vi "Generate Patch Seq Img Core.vi"(0 "tdms file ref":refnum<k34>, 1 "Channel to process":enum16{"Red", "Green"}(ring), 5 "All header parameters":T1={"LOGIN"={"User"="Olympus  20X", "Profile"="", "Software Version"="", "Experiment Date Time"=timestamp(0 s since 1904-01-01)}, "GLOBAL PARAMETERS"={"MicroscopeID"="", "Microscope Type"="", "Objective"="", "Field of View (um)"=0.0, "Fill time (us)"=0.0, "Experiment Type"=enum."In vivo", "Stimuli Trigger"=FALSE, "Speed Logging"=FALSE}, "IMAGING MODES"={"Time Series"=FALSE, "Motor Zstack"=FALSE, "AOL Zstack"=FALSE, "Functional Imaging"=FALSE, "Volume Imaging"=FALSE}, "TIME SERIES"={"Basic Image meta data"={"Wavelength (nm)"=0.0, "# averaged frames"=0.0, "laser power (%)"=0.0, "Pockels"=0.0, "pixel dwell time (us)"=0.0, "pmt 1"=0.0, "pmt 2"=0.0, "back apperture"=0.0, "zoom"=0.0, "field of view"=0.0, "Frame Size"=200, "AOL x centre"=0.0, "AOL y centre"=0.0, "Stage x position"=0.0, "Stage y position"=0.0, "Stage z position"=0.0}, "AOL z"=0.0}, "MOTOR Z-STACK "={"Hdr Basic Image meta data"={"Wavelength (nm)"=0.0, "# averaged frames"=0.0, "laser power (%)"=0.0, "Pockels"=0.0, "pixel dwell time (us)"=0.0, "pmt 1"=0.0, "pmt 2"=0.0, "back apperture"=0.0, "zoom"=0.0, "field of view"=0.0, "Frame Size"=0, "AOL x centre"=0.0, "AOL y centre"=0.0, "Stage x position"=0.0, "Stage y position"=0.0, "Stage z position"=0.0}, "Z Start"=0.0, "Z Stop"=0.0, "No of Planes"=0, "Laser Power (%) at Z Start"=0.0, "Laser Power (%) at Z Stop"=0.0}, "AOL Z-STACK"={"Hdr Basic Image meta data"={"Wavelength (nm)"=0.0, "# averaged frames"=0.0, "laser power (%)"=0.0, "Pockels"=0.0, "pixel dwell time (us)"=0.0, "pmt 1"=0.0, "pmt 2"=0.0, "back apperture"=0.0, "zoom"=0.0, "field of view"=0.0, "Frame Size"=0, "AOL x centre"=0.0, "AOL y centre"=0.0, "Stage x position"=0.0, "Stage y position"=0.0, "Stage z position"=0.0}, "Z Start"=0.0, "Z Stop"=0.0, "No of Planes"=0, "Laser Power (%) at Z Start"=0.0, "Laser Power (%) at Z Stop"=0.0}, "FUNCTIONAL IMAGING"={"Functional Mode"=enum."Point", "Variable Length"=FALSE, "Variable Resolution"=FALSE, "Pockels Modulation"=FALSE, "Stimuli Trigger"=FALSE, "Cool down enabled"=FALSE, "AOL Mode"=enum."Raster", "Plane Mode"=0, "Miniscan Dwell time per pixel (us)"=0.0, "poi dwell time"=0.0, "Number of trials"=0.0, "Number of cycles"=0.0, "Number of pois"=0.0, "Number of miniscans"=0.0, "Number of pixels in miniscan"=0.0, "Rectangle ROI length"=0.0, "Rectangle ROI height"=0.0, "Frame rate (fps)"=0.0, "Acquisition Length"=0.0, "video length (sec)"=0.0, "Stimuli delay (sec)"=0.0, "Cool down time (sec)"=0.0, "Basic Image meta data"={"Wavelength (nm)"=0.0, "# averaged frames"=0.0, "laser power (%)"=0.0, "Pockels"=0.0, "pixel dwell time (us)"=0.0, "pmt 1"=0.0, "pmt 2"=0.0, "back apperture"=0.0, "zoom"=0.0, "field of view"=0.0, "Frame Size"=0, "AOL x centre"=0.0, "AOL y centre"=0.0, "Stage x position"=0.0, "Stage y position"=0.0, "Stage z position"=0.0}, "Z Start (um)"=0.0, "Z Stop (um)"=0.0}, "VOLUME IMAGING"={"Functional Mode"=enum."Point", "Variable Length"=FALSE, "Variable Resolution"=FALSE, "Pockels Modulation"=FALSE, "Stimuli Trigger"=FALSE, "Cool down enabled"=FALSE, "AOL Mode"=enum."Raster", "Plane Mode"=0, "Miniscan Dwell time per pixel (us)"=0.0, "poi dwell time"=0.0, "Number of trials"=0.0, "Number of cycles"=0.0, "Number of pois"=0.0, "Number of miniscans"=0.0, "Number of pixels in miniscan"=0.0, "Rectangle ROI length"=0.0, "Rectangle ROI height"=0.0, "Frame rate (fps)"=0.0, "Acquisition Length"=0.0, "video length (sec)"=0.0, "Stimuli delay (sec)"=0.0, "Cool down time (sec)"=0.0, "Basic Image meta data"={"Wavelength (nm)"=0.0, "# averaged frames"=0.0, "laser power (%)"=0.0, "Pockels"=0.0, "pixel dwell time (us)"=0.0, "pmt 1"=0.0, "pmt 2"=0.0, "back apperture"=0.0, "zoom"=0.0, "field of view"=0.0, "Frame Size"=0, "AOL x centre"=0.0, "AOL y centre"=0.0, "Stage x position"=0.0, "Stage y position"=0.0, "Stage z position"=0.0}, "Z Start (um)"=0.0, "Z Stop (um)"=0.0}, "MOVEMENT CORRECTION"={"Movement Correction"=FALSE, "Axial Reference"=FALSE, "Reference Source"=enum."Green channel", "Full Frame Size"=0.0, "Reference Field of View"=0.0, "Reference Zoom"=0.0, "Reference dwell time (us)"=0.0, "Reference X Pixels"=0.0, "Reference Y Pixels"=0.0, "Number of Z lines"=0.0, "Size of Z pixels"=0.0, "Axial Pixels"=0.0, "Ignore Z lines"=0.0, "Reference Scan Cycles"=0.0, "Reference Threshold XY"=0.0, "Reference Threshold Z"=0.0, "Reference Average XY"=0.0, "Reference Average Z"=0.0, "Proportional Scale"=0.0, "Integral Scale"=0.0, "Proportional Scale Z"=0.0, "Integral Scale Z"=0.0, "Diff Threshold"=0.0, "Diff Threshold Z"=0.0, "Sliding Average"=FALSE, "Reference count reset enabled"=FALSE, "Scan Interval (ms)"=0.0, "Ref Plot Refresh Rate (ms)"=0.0}, "CALIBRATION"={"Pockels Calibration File"=path "", "Calibration_ini file"=path "", "Setup_ini file"=path ""}, "STATISTICS"={"Z-stack duration (sec)"=0.0, "Number of acquired data-points"=0.0, "Acquisition time (ms)"=0.0, "Number of acquired frames"=0.0, "Intertrial times"=[]}, "BIOLOGY INFORMATION"={"Animal Code or Name"="", "Animal DoB"="", "Animal Age"="", "Animal Sex"="", "Animal Weight"="", "Date of Injection"="", "Date of Implant"="", "Site of Injection"="", "Animal Ear Notch"="", "AAV constructs"="", "Genetic background"="", "Optical reporter"="", "Region of brain imaged"="", "Other \ncomments"=""}, "Calibration Data"={"Objective Name"="", "Calibration Wavelength"=0.0, "Sum X"=0.0, "Sum Y"=0.0, "Diff X"=0.0, "Diff Y"=0.0, "Distortion Correction"=0.0, " Z norm to um Scaling"=0.0, " X norm to um Scaling"=0.0}} {"VOLUME IMAGING"."Plane Mode" items=["XY Plane", "XZ Plane", "YZ Plane", "arbitraryplane"]; "VOLUME IMAGING"."Basic Image meta data"."Frame Size" items=["100X100"=100, "128X128"=128, "200X200"=200, "256X256"=256, "512X512"=512, "1024x1024"=1024, "2048x2048"=2048]; "AOL Z-STACK"."Hdr Basic Image meta data"."Frame Size" items=["100X100"=100, "128X128"=128, "200X200"=200, "256X256"=256, "512X512"=512, "1024x1024"=1024, "2048x2048"=2048]; "MOTOR Z-STACK"."Hdr Basic Image meta data"."Frame Size" items=["100X100"=100, "128X128"=128, "200X200"=200, "256X256"=256, "512X512"=512, "1024x1024"=1024, "2048x2048"=2048]; "FUNCTIONAL IMAGING"."Plane Mode" items=["XY Plane", "XZ Plane", "YZ Plane", "arbitraryplane"]; "FUNCTIONAL IMAGING"."Basic Image meta data"."Frame Size" items=["100X100"=100, "128X128"=128, "200X200"=200, "256X256"=256, "512X512"=512, "1024x1024"=1024, "2048x2048"=2048]; "TIME SERIES"."Basic Image meta data"."Frame Size" items=["100X100"=100, "128X128"=128, "200X200"=200, "256X256"=256, "512X512"=512, "1024x1024"=1024, "2048x2048"=2048]}, 7 "TDMS file path & name":path=path "C:/Users/Theo/Desktop/Datasets/140401_17_44_08-rig 3 debugging/Functional imaging TDMS data files/001.tdms", 9 "Patch Image Folder":path[](array[path]), 11 "error in (no error)":errorcluster, 13 "TIFF file handles":i32[](array[numeric]), 14 "Trial Number":i32) -> (4 "tdms file out":refnum<k34>, 15 "error out":errorcluster)   [LabVIEW 2020]
uses:
  <vilib>/vision/NI_Vision_Development_Module.lvlib
  Typedefs/Channel Selector.ctl
  Globals/gl_funct TIFF export globals.vi
  Typedefs/Frame Size.ctl
  Typedefs/AOL modes.ctl
  Typedefs/Plane Mode.ctl
  User Interface/Visualisation/Functional Imaging Viewer/SubVIs/Experiment header interface/Typedefs/Header parameters cluster-ALL.ctl
  User Interface/Visualisation/Functional Imaging Viewer/SubVIs/Experiment header interface/Typedefs/Header subclusters/Header params -Login.ctl
  User Interface/Misc/Experiment Type.ctl
  User Interface/Visualisation/Functional Imaging Viewer/SubVIs/Experiment header interface/Typedefs/Header subclusters/Header params-Global Parameters.ctl
  User Interface/Visualisation/Functional Imaging Viewer/SubVIs/Experiment header interface/Typedefs/Header subclusters/Header params-Imaging Modes.ctl
  User Interface/Visualisation/Functional Imaging Viewer/SubVIs/Experiment header interface/Typedefs/Header subclusters/Header params-Basic image meta data.ctl
  User Interface/Visualisation/Functional Imaging Viewer/SubVIs/Experiment header interface/Typedefs/Header subclusters/Header params-Time Series.ctl
  Typedefs/Functional Mode.ctl
  User Interface/Visualisation/Functional Imaging Viewer/SubVIs/Experiment header interface/Typedefs/Header subclusters/Header params-Functional Imaging.ctl
  Typedefs/Reference source.ctl
  User Interface/Visualisation/Functional Imaging Viewer/SubVIs/Experiment header interface/Typedefs/Header subclusters/Header params-Movement correction.ctl
  User Interface/Visualisation/Functional Imaging Viewer/SubVIs/Experiment header interface/Typedefs/Header subclusters/Header params-Calibration Setup.ctl
  User Interface/Visualisation/Functional Imaging Viewer/SubVIs/Experiment header interface/Typedefs/Header subclusters/Header params-statistics.ctl
  User Interface/Misc/Biology Information.ctl
  User Interface/Visualisation/Functional Imaging Viewer/SubVIs/Experiment header interface/Typedefs/Header subclusters/Header params-Motor Z-stack.ctl
  User Interface/Visualisation/Functional Imaging Viewer/SubVIs/Experiment header interface/Typedefs/Header subclusters/Header params-AOL Z-stack.ctl
  User Interface/Visualisation/Functional Imaging Viewer/SubVIs/Experiment header interface/Typedefs/Header subclusters/Header params-calibration data.ctl
panel:
  out "Loop time (ms)":u32
  # "Re-entrant"
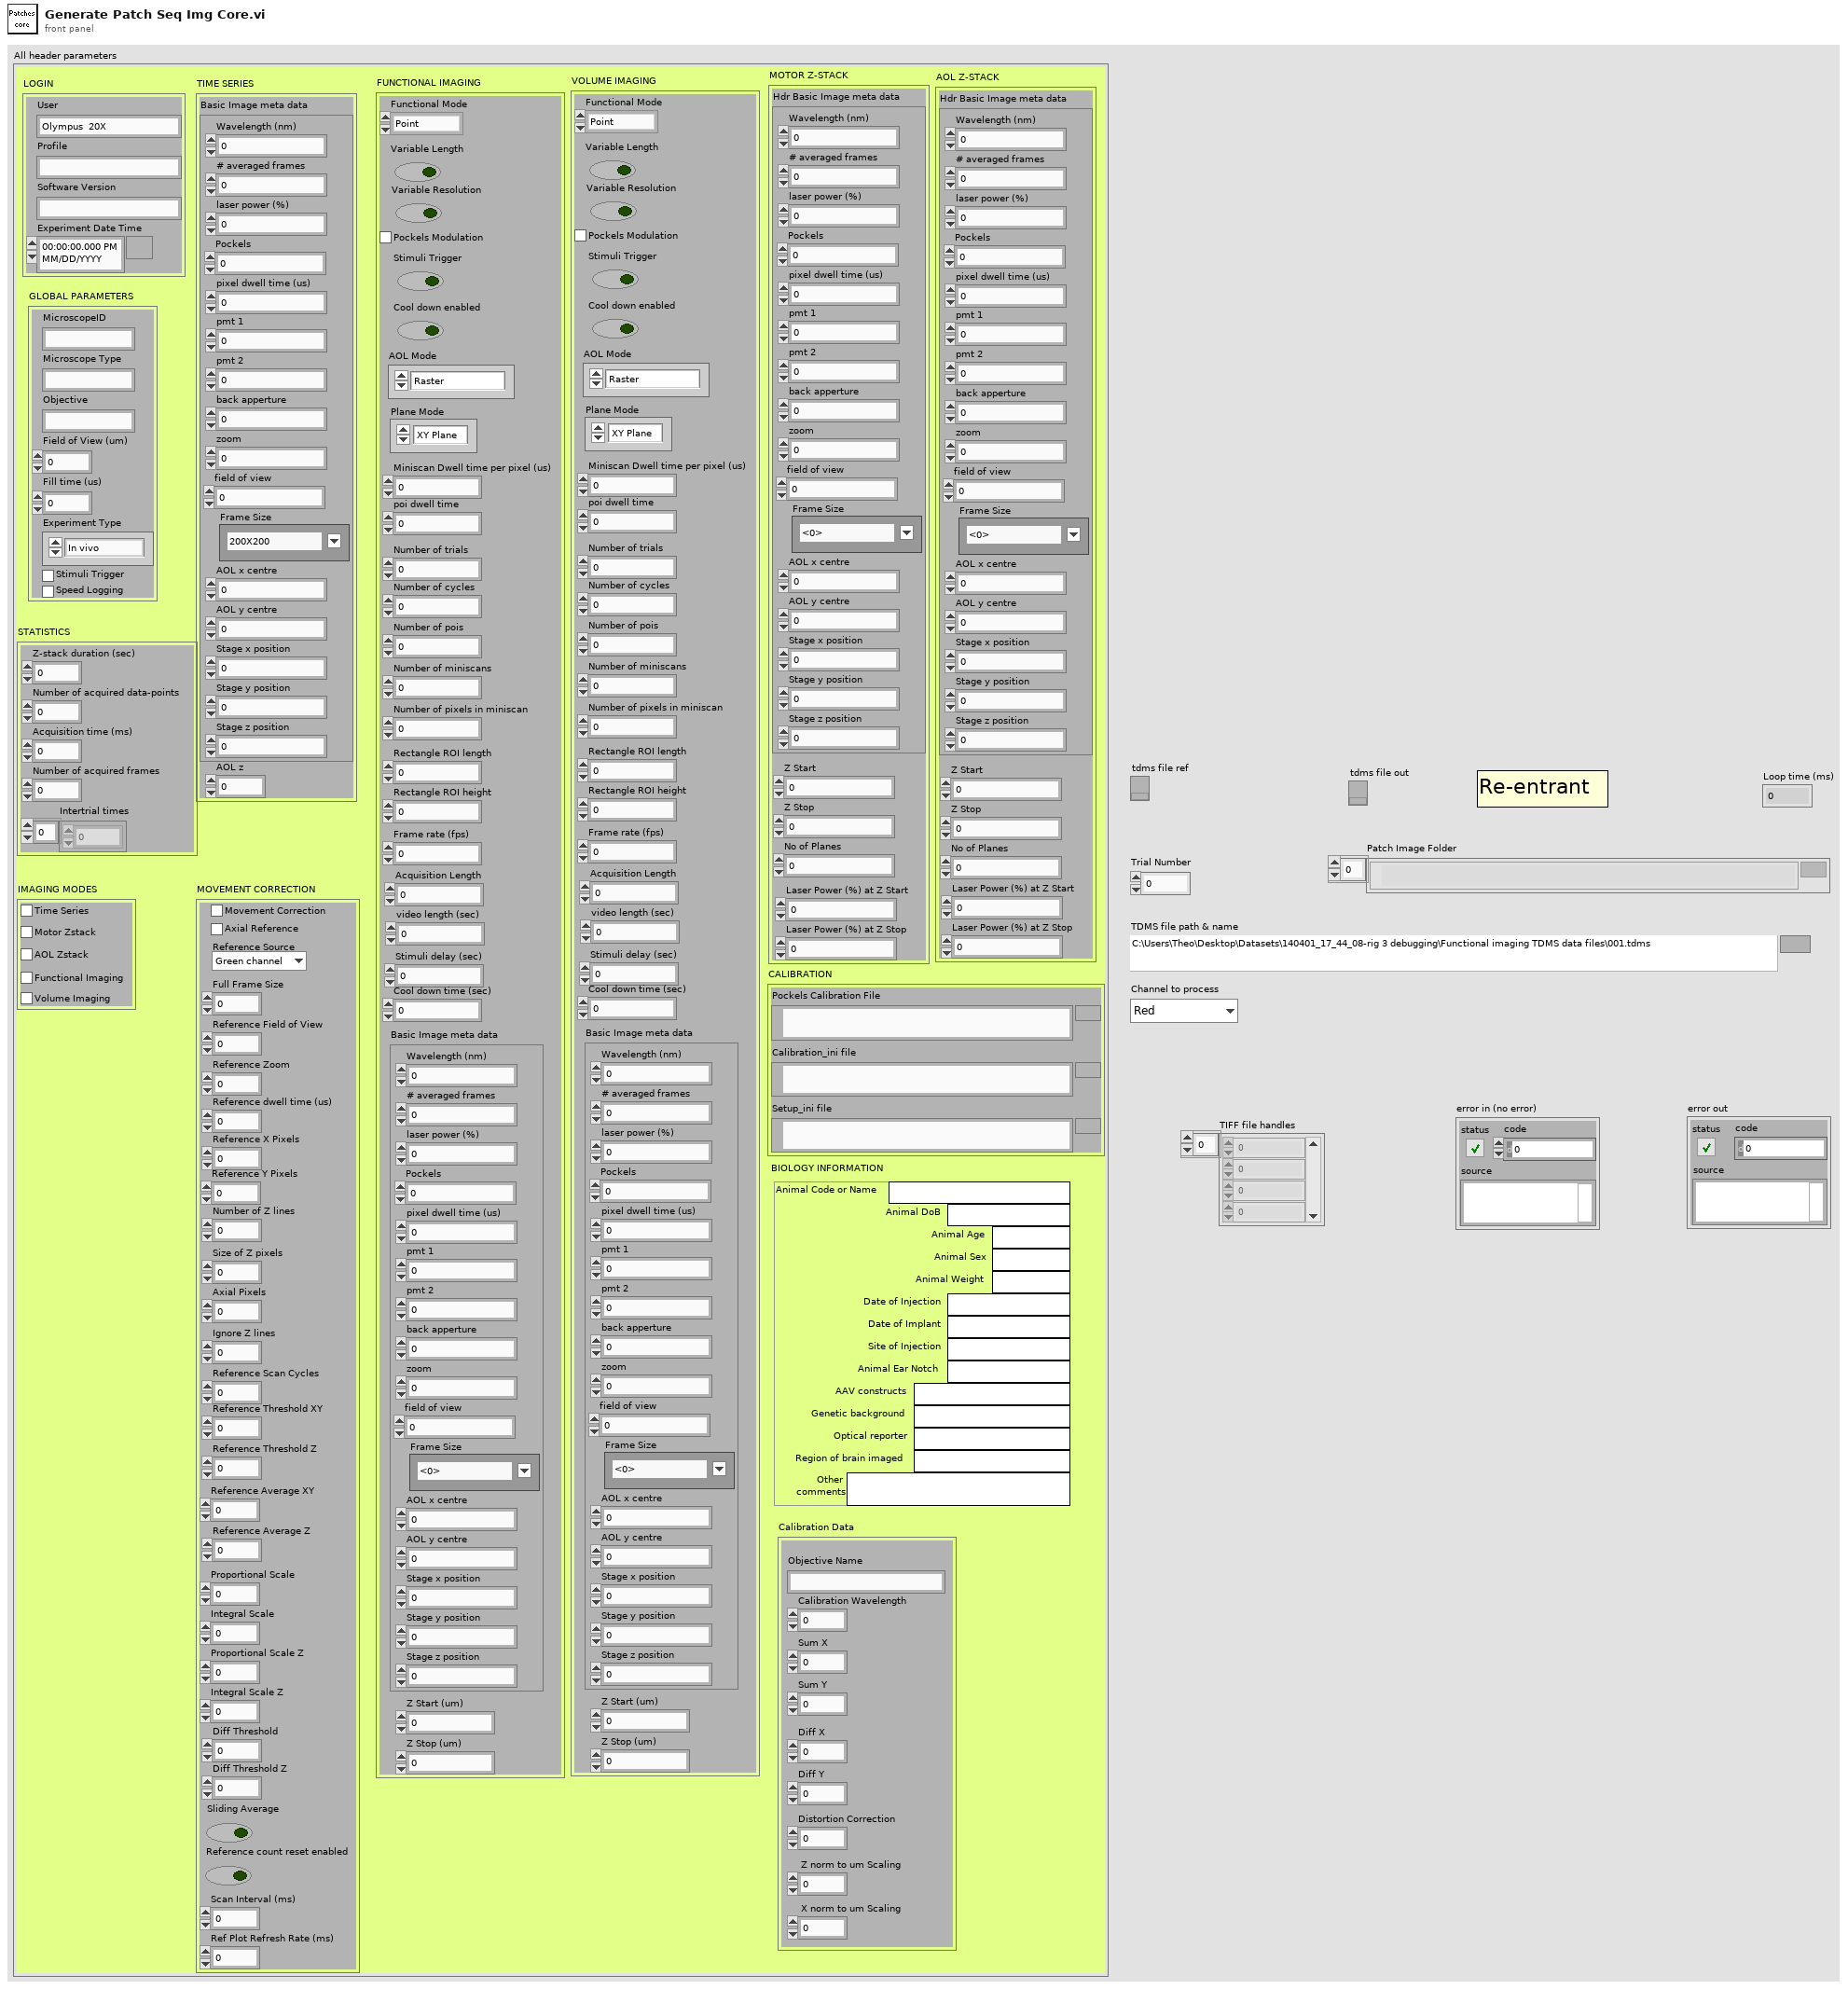
[diagram p1: front panel]
types:
  T1 = typedef "Header parameters cluster-ALL.ctl" = cluster{"LOGIN":T2, "GLOBAL PARAMETERS":T3, "IMAGING MODES":T5, "TIME SERIES":T6, "MOTOR Z-STACK ":T9, "AOL Z-STACK":T10, "FUNCTIONAL IMAGING":T11, "VOLUME IMAGING":T11, "MOVEMENT CORRECTION":T15, "CALIBRATION":T17, "STATISTICS":T18, "BIOLOGY INFORMATION":T19, "Calibration Data":T20}
  T2 = typedef "Header params -Login.ctl" = cluster{"User":string, "Profile":string, "Software Version":string, "Experiment Date Time":timestamp}
  T3 = typedef "Header params-Global Parameters.ctl" = cluster{"MicroscopeID":string, "Microscope Type":string, "Objective":string, "Field of View (um)":dbl, "Fill time (us)":dbl, "Experiment Type":T4, "Stimuli Trigger":bool, "Speed Logging":bool}
  T4 = typedef "Experiment Type.ctl" = enum16{"In vivo", "In vitro", "Testing", "Calibration", "Other"}
  T5 = typedef "Header params-Imaging Modes.ctl" = cluster{"Time Series":bool, "Motor Zstack":bool, "AOL Zstack":bool, "Functional Imaging":bool, "Volume Imaging":bool}
  T6 = typedef "Header params-Time Series.ctl" = cluster{"Basic Image meta data":T7, "AOL z":dbl}
  T7 = typedef "Header params-Basic image meta data.ctl" = cluster{"Wavelength (nm)":dbl, "# averaged frames":dbl, "laser power (%)":dbl, "Pockels":dbl, "pixel dwell time (us)":dbl, "pmt 1":dbl, "pmt 2":dbl, "back apperture":dbl, "zoom":dbl, "field of view":dbl, "Frame Size":T8, "AOL x centre":dbl, "AOL y centre":dbl, "Stage x position":dbl, "Stage y position":dbl, "Stage z position":dbl}
  T8 = typedef "Frame Size.ctl" = u16
  T9 = typedef "Header params-Motor Z-stack.ctl" = cluster{"Hdr Basic Image meta data":T7, "Z Start":dbl, "Z Stop":dbl, "No of Planes":i32, "Laser Power (%) at Z Start":dbl, "Laser Power (%) at Z Stop":dbl}
  T10 = typedef "Header params-AOL Z-stack.ctl" = cluster{"Hdr Basic Image meta data":T7, "Z Start":dbl, "Z Stop":dbl, "No of Planes":i32, "Laser Power (%) at Z Start":dbl, "Laser Power (%) at Z Stop":dbl}
  T11 = typedef "Header params-Functional Imaging.ctl" = cluster{"Functional Mode":T12, "Variable Length":bool, "Variable Resolution":bool, "Pockels Modulation":bool, "Stimuli Trigger":bool, "Cool down enabled":bool, "AOL Mode":T13, "Plane Mode":T14, "Miniscan Dwell time per pixel (us)":dbl, "poi dwell time":dbl, "Number of trials":dbl, "Number of cycles":dbl, "Number of pois":dbl, "Number of miniscans":dbl, "Number of pixels in miniscan":dbl, "Rectangle ROI length":dbl, "Rectangle ROI height":dbl, "Frame rate (fps)":dbl, "Acquisition Length":dbl, "video length (sec)":dbl, "Stimuli delay (sec)":dbl, "Cool down time (sec)":dbl, "Basic Image meta data":T7, "Z Start (um)":dbl, "Z Stop (um)":dbl}
  T12 = typedef "Functional Mode.ctl" = enum16{"Point", "Line", "Patch", "Plane", "Volume"}
  T13 = typedef "AOL modes.ctl" = enum16{"Raster", "Structural", "Pointing", "Mini Scan", "Alignment"}
  T14 = typedef "Plane Mode.ctl" = u16
  T15 = typedef "Header params-Movement correction.ctl" = cluster{"Movement Correction":bool, "Axial Reference":bool, "Reference Source":T16, "Full Frame Size":dbl, "Reference Field of View":dbl, "Reference Zoom":dbl, "Reference dwell time (us)":dbl, "Reference X Pixels":dbl, "Reference Y Pixels":dbl, "Number of Z lines":dbl, "Size of Z pixels":dbl, "Axial Pixels":dbl, "Ignore Z lines":dbl, "Reference Scan Cycles":dbl, "Reference Threshold XY":dbl, "Reference Threshold Z":dbl, "Reference Average XY":dbl, "Reference Average Z":dbl, "Proportional Scale":dbl, "Integral Scale":dbl, "Proportional Scale Z":dbl, "Integral Scale Z":dbl, "Diff Threshold":dbl, "Diff Threshold Z":dbl, "Sliding Average":bool, "Reference count reset enabled":bool, "Scan Interval (ms)":dbl, "Ref Plot Refresh Rate (ms)":dbl}
  T16 = typedef "Reference source.ctl" = enum16{"Green channel", "Red channel"}
  T17 = typedef "Header params-Calibration Setup.ctl" = cluster{"Pockels Calibration File":path, "Calibration_ini file":path, "Setup_ini file":path}
  T18 = typedef "Header params-statistics.ctl" = cluster{"Z-stack duration (sec)":dbl, "Number of acquired data-points":dbl, "Acquisition time (ms)":dbl, "Number of acquired frames":dbl, "Intertrial times":dbl[]}
  T19 = typedef "Biology Information.ctl" = cluster{"Animal Code or Name":string, "Animal DoB":string, "Animal Age":string, "Animal Sex":string, "Animal Weight":string, "Date of Injection":string, "Date of Implant":string, "Site of Injection":string, "Animal Ear Notch":string, "AAV constructs":string, "Genetic background":string, "Optical reporter":string, "Region of brain imaged":string, "Other \ncomments":string}
  T20 = typedef "Header params-calibration data.ctl" = cluster{"Objective Name":string, "Calibration Wavelength":dbl, "Sum X":dbl, "Sum Y":dbl, "Diff X":dbl, "Diff Y":dbl, "Distortion Correction":dbl, " Z norm to um Scaling":dbl, " X norm to um Scaling":dbl}
  T21 = typedef "Funct TIFF exporter ctrl refs.ctl" = cluster{"This VI":refnum<vi>, "Current Experiment":refnum<vi>, "Imaging protocol":refnum<vi>, "Predominant ROI type":refnum<vi>, "Patches in Experiment":refnum<vi>, "Folder Path":refnum<vi>, "Export":refnum<vi>, "Trial number":refnum<vi>, "Output TIFF type":refnum<vi>}
  T22 = typedef "Exported TIFF type.ctl" = enum16{"One multi-page TIFF file for each rectangle", "Individual TIFF files"}
  T23 = typedef "Channel Selector.ctl" = enum16{"Red Channel", "Green Channel", "Blended"}
  T24 = cluster{"Number of cycles":i32, "number of planes":i32, "number of miniscans in a Plane":i32, "number of pixels in a miniscan":i32}
  T25 = typedef "Image Type" = u32
  T26 = typedef "IMAQ Image.ctl" = refnum<image>
  T27 = typedef "IMAQ AVI2 Refnum.ctl" = refnum<k20>
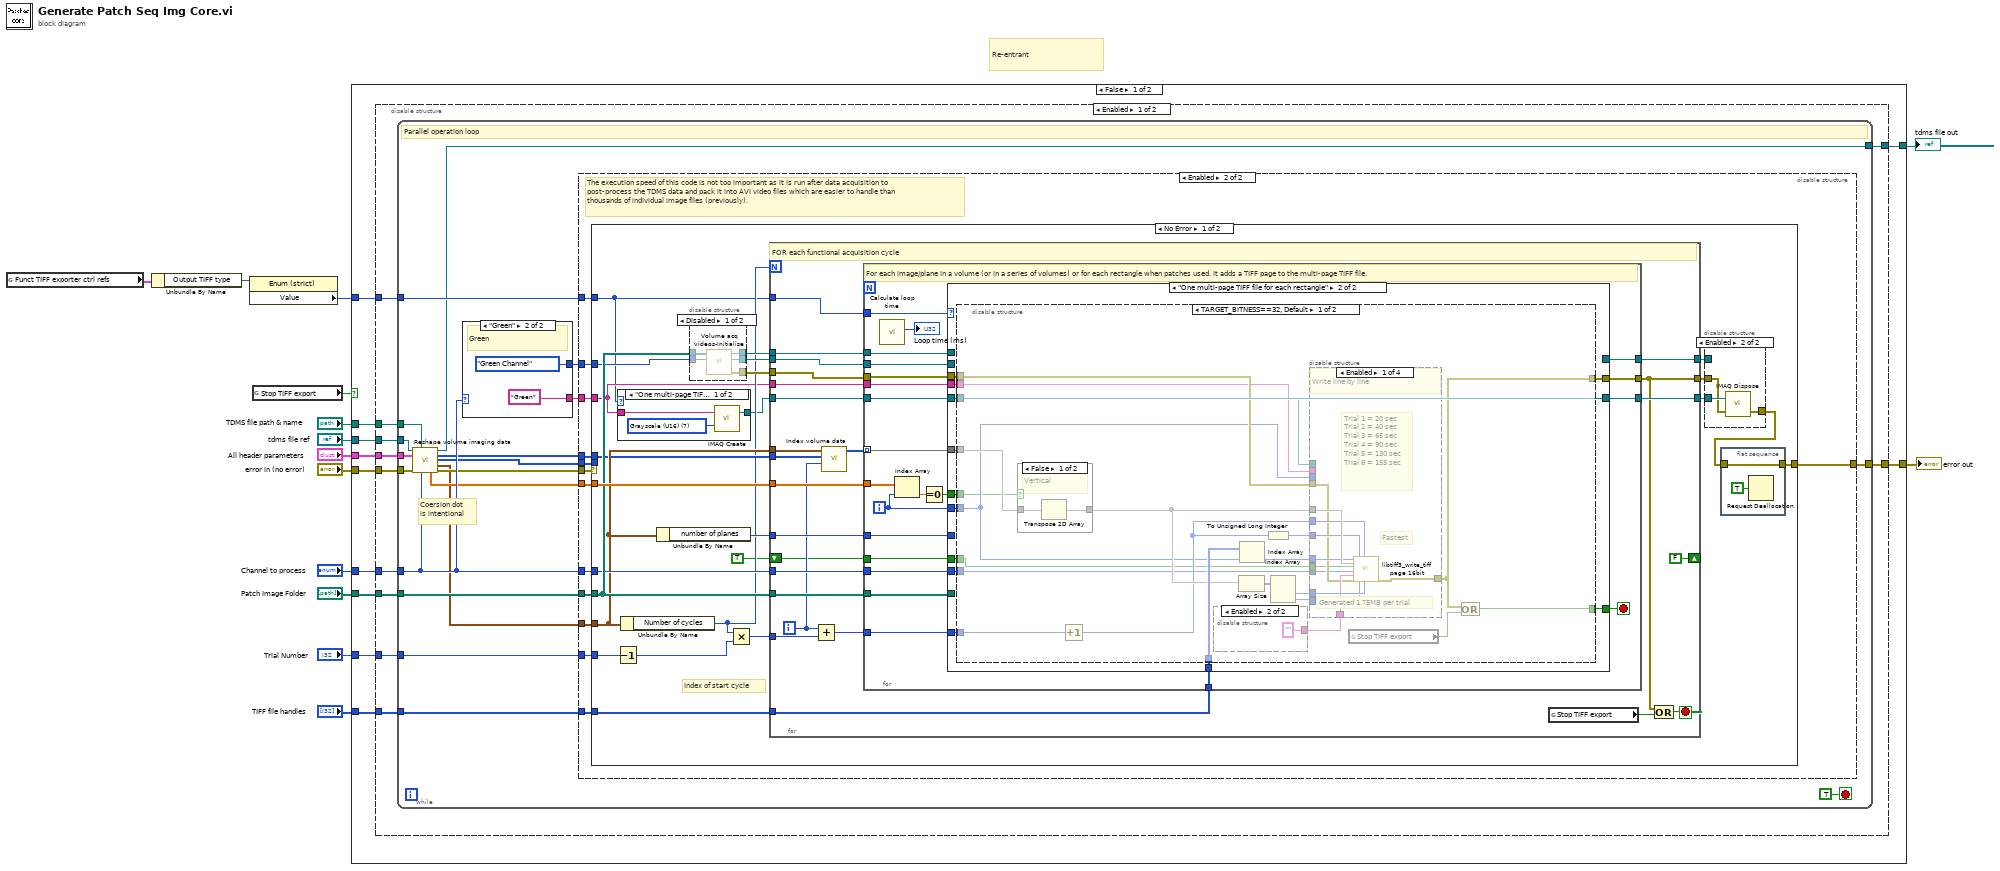
[diagram p0: block diagram]
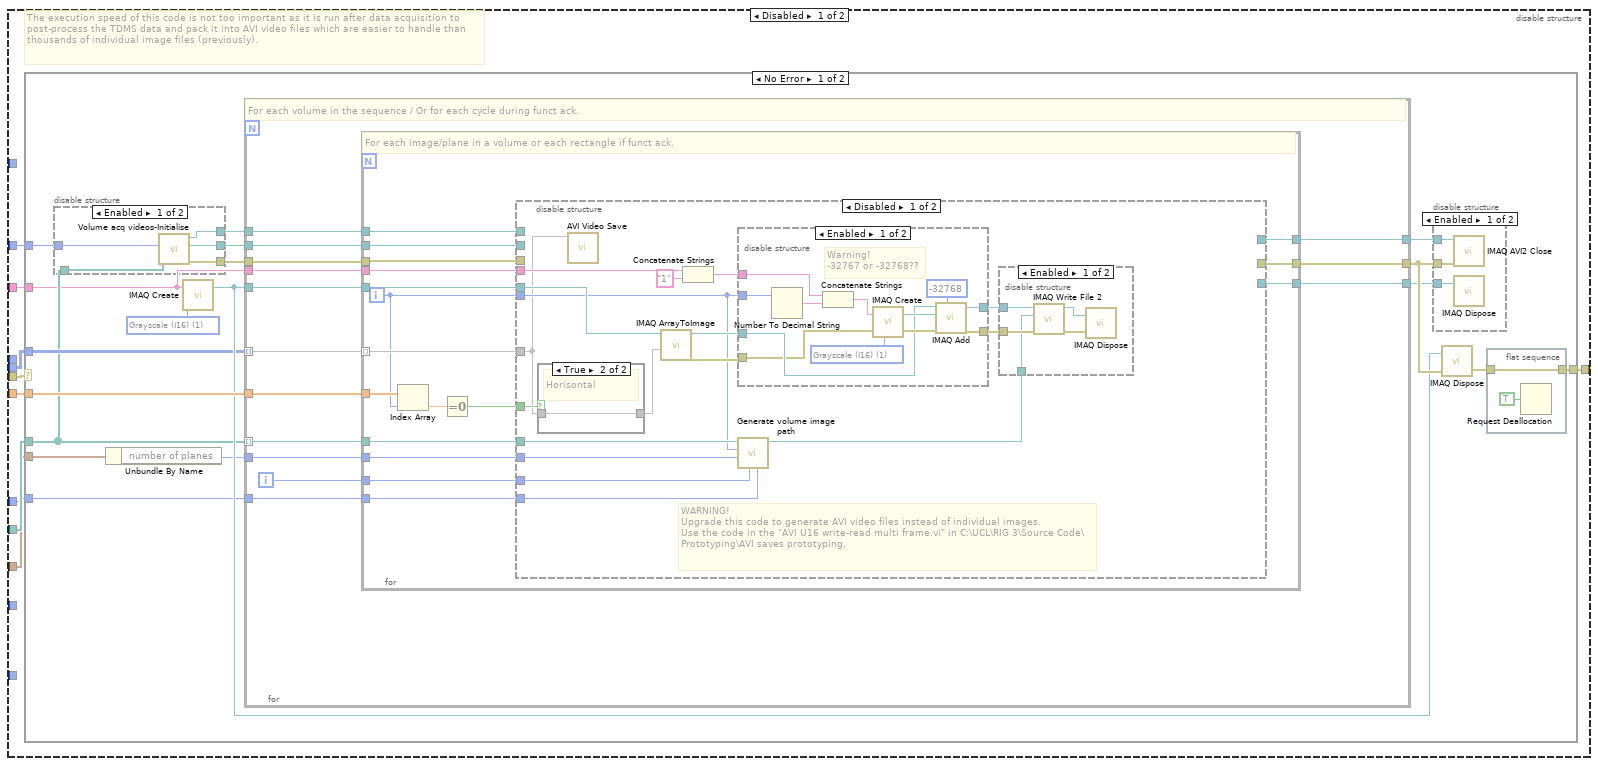
[diagram p2: hidden frame]
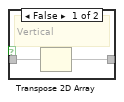
[diagram p5: hidden frame]
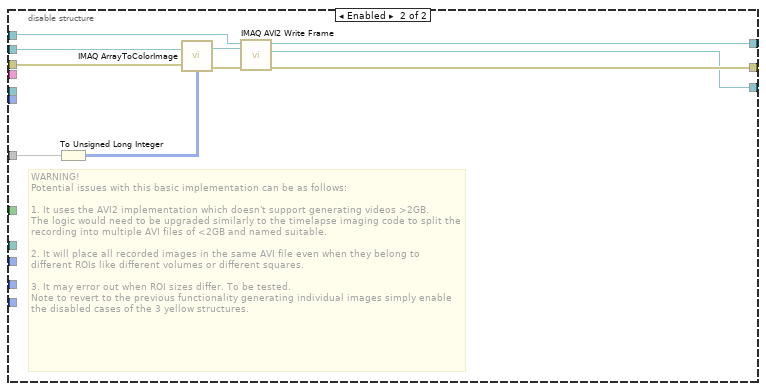
[diagram p8: hidden frame]
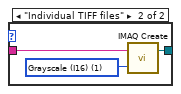
[diagram p10: hidden frame]
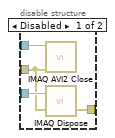
[diagram p12: hidden frame]
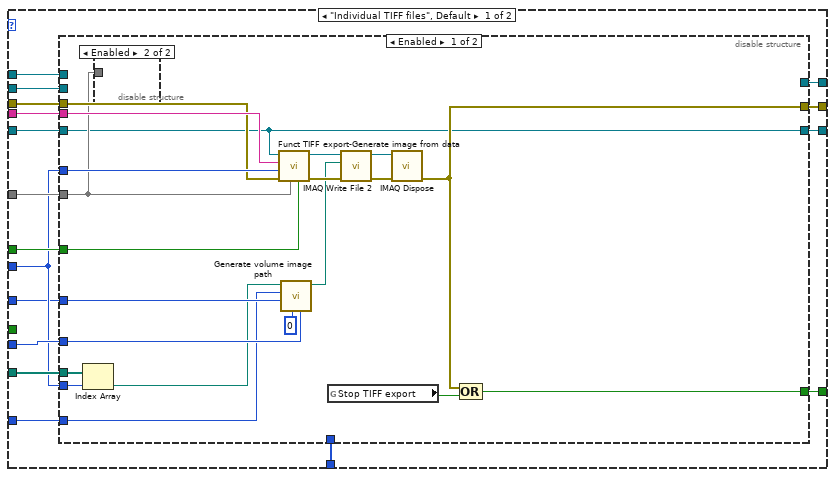
[diagram p13: hidden frame]
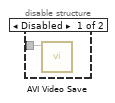
[diagram p14: hidden frame]
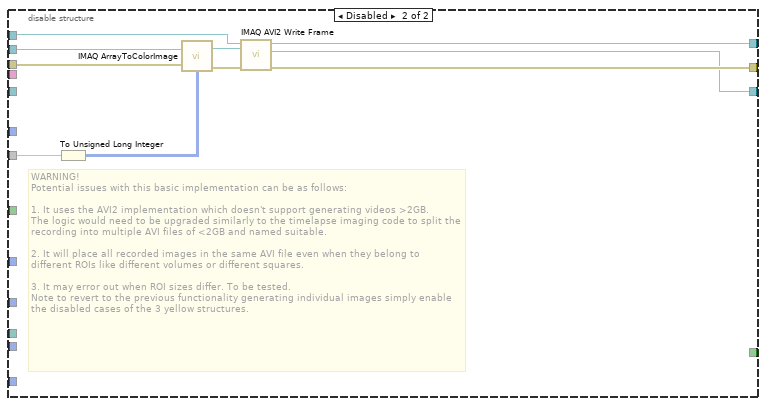
[diagram p15: hidden frame]
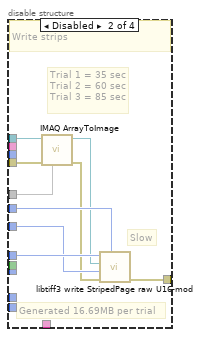
[diagram p16: hidden frame]
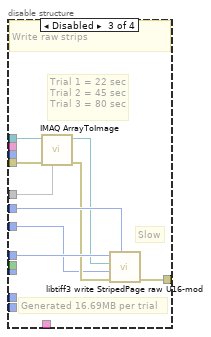
[diagram p17: hidden frame]
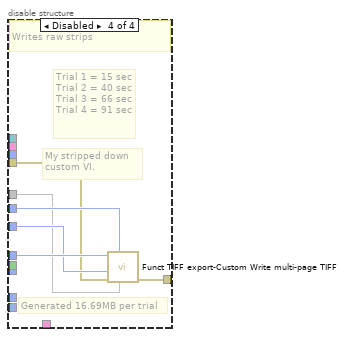
[diagram p18: hidden frame]
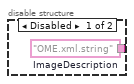
[diagram p19: hidden frame]
diagram:
  # "Re-entrant"
  n1 = global read "gl_funct TIFF export globals.vi" "Funct TIFF exporter ctrl refs"() -> (w6:T21)
  n2 = Unbundle By Name(w6) -> ("Output TIFF type"=w7:refnum<vi>)
  n3 = property on="Property Node" class="Enum (strict)"(reference=w7) -> ("Value"=w5:T22)  [unwired: 1 in, 2 out]
  n4 = global read "gl_funct TIFF export globals.vi" "Stop TIFF export"() -> (w10:bool)
  n5 = case shown="False" w10 {
    tunnel: [w25 w540] -> w14
    tunnel: "error in (no error)" -> [w24 w540]
    tunnel: "Channel to process" -> [w23 _]
    tunnel: "Patch Image Folder" -> [w22 _]
    tunnel: "Trial Number" -> [w21 _]
    tunnel: "TIFF file handles" -> [w20 _]
    tunnel: w5 -> [w19 _]
    tunnel: "tdms file ref" -> [w18 w539]
    tunnel: "All header parameters" -> [w17 _]
    tunnel: "TDMS file path & name" -> [w16 _]
    tunnel: [w15 w539] -> w1
    frame False {
      n6 = disable-structure shown="Enabled" {
        disable-tunnel: [w36 w411] -> w25
        disable-tunnel: w22 -> [w35 w410]
        disable-tunnel: w24 -> [w34 w409]
        disable-tunnel: w23 -> [w33 w408]
        disable-tunnel: w21 -> [w32 _]
        disable-tunnel: w20 -> [w31 _]
        disable-tunnel: w19 -> [w30 _]
        disable-tunnel: w18 -> [w29 w406]
        disable-tunnel: w17 -> [w28 w405]
        disable-tunnel: w16 -> [w27 w407]
        disable-tunnel: [w26 w404] -> w15
        frame Enabled {
          n7 = while {
            tunnel: [w55] -> w36
            tunnel: w35 -> [w54]
            tunnel: w34 -> [w53]
            tunnel: w33 -> [w52]
            tunnel: w32 -> [w51]
            tunnel: w31 -> [w50]
            tunnel: w30 -> [w49]
            tunnel: w29 -> [w38]
            tunnel: w28 -> [w41]
            tunnel: w27 -> [w40]
            tunnel: [w39] -> w26
            stop <- TRUE stop-if-true
            # "Coersion dot\nis intentional"
            # "Parallel operation loop"
            n8 = call "Reshape volume imaging data.vi"("tdms file ref"=w38, "TDMS file path & name"=w40, "All header parameters"=w41, "error in (no error)"=w53, "Channel to process"=w52) -> ("tdms file out"=w39:refnum<k34>, "Single channel data"=w43:u16[], "Channel 4D data"=w42:u16[][][][], "Volumetric parameters"=w44:T24, "Angles (deg)"=w45:dbl[], "error out"=w47:errorcluster)  [unwired: 5 in]
            n9 = case shown="\"Green\"" w52 {
              tunnel: ["Red" ("Image Name") "Green" ("Image Name")] -> w48
              tunnel: [Channel_Selector."Red Channel" ("Channel") Channel_Selector."Green Channel" ("Channel")] -> w46
              frame "Red", Default {
                # "Red"
              }
              frame "Green" {
                # "Green"
              }
            }
            n10 = disable-structure shown="Enabled" {
              disable-tunnel: [w64 w186] -> w55
              disable-tunnel: w54 -> [w63 w185]
              disable-tunnel: w48 -> [w62 w184]
              disable-tunnel: w42 -> [w61 w183]
              disable-tunnel: w47 -> [w60 w182]
              disable-tunnel: w46 -> [w59 w181]
              disable-tunnel: w45 -> [w58 w180]
              disable-tunnel: w52 -> [w57 w179]
              disable-tunnel: w44 -> [w56 w178]
              disable-tunnel: w43 -> [_ w177]
              disable-tunnel: w51 -> [_ w175]
              disable-tunnel: w50 -> [_ w176]
              disable-tunnel: w49 -> [_ w174]
              frame Disabled {
                # "The execution speed of this code is not too important as it is run after data acquisition to post-process the TDMS data and pack it into AVI video files which are easier to handle than thousands of individual image files (previously)."
                n11 = case shown="No Error" w60 {
                  selector: w60 -> [_ w173]
                  tunnel: [w68 w173] -> w64
                  tunnel: w58 -> [w82 _]
                  tunnel: w61 -> [w74 _]
                  tunnel: w56 -> [w65 _]
                  tunnel: w63 -> [w71 _]
                  tunnel: w62 -> [w70 _]
                  tunnel: w57 -> [w67 _]
                  tunnel: w59 -> [w66 _]
                  frame No Error {
                    w73 = T25 1 items=["Grayscale (U8)", "Grayscale (I16)", "Grayscale (SGL)", "Complex (CSG)", "RGB (U32)", "HSL (U32)", "RGB (U64)", "Grayscale (U16)"] ("Image Type")
                    n12 = disable-structure "Diagram Disable Structure" shown="Enabled" {
                      disable-tunnel: [w89 _] -> w75
                      disable-tunnel: [w88 _] -> w76
                      disable-tunnel: [w87 _] -> w77
                      disable-tunnel: w71 -> [w86 _]
                      disable-tunnel: w66 -> [w85 _]
                      frame Enabled {
                        n13 = call "Volume acq videos-Initialise.vi"("Channel"=w85, "created path"=w86) -> ("error out"=w89:errorcluster, "Temp Image"=w88:T26, "Refnum out"=w87:T27)  [unwired: 7 in]
                      }
                      frame Disabled {
                      }
                    }
                    n14 = Unbundle By Name(w65) -> ("number of planes"=w72:i32)
                    n15 = call "IMAQ Create"("Image Name"=w70, "Image Type"=w73) -> ("New Image"=w80:T26)  [unwired: 3 in, 1 out]
                    n16 = for {
                      tunnel: w74 -> [w106] mode=indexing
                      tunnel: w80 -> [w105]
                      tunnel: w71 -> [w104] mode=indexing
                      tunnel: w72 -> [w102]
                      tunnel: w76 -> [w101]
                      tunnel: w77 -> [w100]
                      tunnel: w75 -> [w99]
                      tunnel: [w98] -> w81
                      tunnel: [w97] -> w78
                      tunnel: [w96] -> w79
                      tunnel: w82 -> [w95]
                      tunnel: w70 -> [w94]
                      tunnel: w67 -> [w93]
                      i -> [w103]
                      # "For each volume in the sequence / Or for each cycle during funct ack."
                      n17 = for {
                        tunnel: w106 -> [w110] mode=indexing
                        tunnel: w105 -> [w123]
                        tunnel: w104 -> [w122]
                        tunnel: w103 -> [w121]
                        tunnel: w102 -> [w120]
                        tunnel: w101 -> [w118]
                        tunnel: w100 -> [w119]
                        tunnel: w99 -> [w117]
                        tunnel: [w116] -> w98
                        tunnel: [w115] -> w97
                        tunnel: [w114] -> w96
                        tunnel: w95 -> [w109]
                        tunnel: w94 -> [w112]
                        tunnel: w93 -> [w111]
                        i -> [w108]
                        # "For each image/plane in a volume or each rectangle if funct ack."
                        n18 = Index Array(array=w109, index=w108) -> (element=w107:dbl)
                        n19 = Equal To 0?(x=w107) -> (x = 0?=w113:bool)
                        n20 = disable-structure shown="Disabled" {
                          disable-tunnel: w123 -> [w140 _]
                          disable-tunnel: w122 -> [w135 _]
                          disable-tunnel: w121 -> [w133 _]
                          disable-tunnel: w120 -> [w132 _]
                          disable-tunnel: w108 -> [w131 _]
                          disable-tunnel: w119 -> [_ w169]
                          disable-tunnel: w118 -> [_ w168]
                          disable-tunnel: w117 -> [_ w167]
                          disable-tunnel: [_ w166] -> w116
                          disable-tunnel: [_ w165] -> w115
                          disable-tunnel: [_ w164] -> w114
                          disable-tunnel: w113 -> [w130 _]
                          disable-tunnel: w110 -> [w125 w163]
                          disable-tunnel: w112 -> [w128 _]
                          disable-tunnel: w111 -> [w124 _]
                          frame Disabled {
                            # "WARNING!\nUpgrade this code to generate AVI video files instead of individual images.\nUse the code in the \"AVI U16 write-read multi frame.vi\" in C:\\UCL\\RIG 3\\Source Code\\Prototyping\\AVI saves prototyping."
                            n21 = case shown="True" w130 {
                              tunnel: w125 -> [w142 w143]
                              tunnel: [w141 w143] -> w129
                              frame False {
                                # "Vertical"
                                n22 = Transpose 2D Array(2D array=w142) -> (transposed array=w141:u16[][])
                              }
                              frame True {
                                # "Horisontal"
                              }
                            }
                            n23 = call "AVI Video Save.vi"("Image Pixels"=w125) -> ()  [unwired: 9 in, 2 out]
                            n24 = call "IMAQ ArrayToImage"("Image Pixels (I16)"=w129, "Image"=w140) -> ("error out"=w136:errorcluster, "Image Out"=w139:T26)  [unwired: 8 in]
                            n25 = Concatenate Strings(w128, "1" ("string")) -> (w126:string)
                            n26 = call "Generate volume image path.vi"("Channel to process"=w124, "Volume index"=w133, "Number of planes"=w132, "Plane index (within its volume)"=w131, "Folder path"=w135) -> ("File path"=w134:path)  [unwired: 5 in, 1 out]
                            n27 = disable-structure shown="Enabled" {
                              disable-tunnel: w131 -> [w154 _]
                              disable-tunnel: w139 -> [w153 w162]
                              disable-tunnel: [w152 w162] -> w138
                              disable-tunnel: [w150 w161] -> w137
                              disable-tunnel: w136 -> [w151 w161]
                              disable-tunnel: w126 -> [w149 _]
                              frame Enabled {
                                w156 = T25 1 items=["Grayscale (U8)", "Grayscale (I16)", "Grayscale (SGL)", "Complex (CSG)", "RGB (U32)", "HSL (U32)", "RGB (U64)"] ("Image Type")
                                # "Warning!\n-32767 or -32768??"
                                n28 = Number To Decimal String(number=w154) -> (decimal integer string=w157:string)  [unwired: 1 in]
                                n29 = Concatenate Strings(w149, w157) -> (w158:string)
                                n30 = call "IMAQ Create"("Image Name"=w158, "Image Type"=w156, "error in (no error)"=w151) -> ("New Image"=w159:T26, "error out"=w160:errorcluster)  [unwired: 2 in]
                                n31 = call "IMAQ Add"("Image Src A"=w153, "Constant"=i16 -32768, "Image Dst"=w159, "error in (no error)"=w160) -> ("Image Dst Out"=w152:T26, "error out"=w150:errorcluster)  [unwired: 3 in]
                              }
                              frame Disabled {
                              }
                            }
                            n32 = disable-structure shown="Enabled" {
                              disable-tunnel: w138 -> [w146 _]
                              disable-tunnel: w137 -> [w145 _]
                              disable-tunnel: w134 -> [w144 _]
                              frame Enabled {
                                n33 = call-poly "IMAQ Write File 2"("error in (no error)"=w145, "File Path"=w144, "Image"=w146) -> ("error out"=w148:errorcluster, "Image Out (duplicate)"=w147:T26)  [unwired: 7 in]
                                n34 = call "IMAQ Dispose"("Image"=w147, "error in (no error)"=w148) -> ()  [unwired: 4 in, 1 out]
                              }
                              frame Disabled {
                              }
                            }
                          }
                          frame Enabled {
                            # "WARNING!\nPotential issues with this basic implementation can be as follows:\n\n1. It uses the AVI2 implementation which doesn't support generating videos >2GB. \nThe logic would need to be upgraded similarly to the timelapse imaging code to split the recording into multiple AVI files of <2GB and named suitable.\n\n2. It will place all recorded images in the same AVI file even when they belong to different ROIs like different volumes or different squares.\n\n3. It may error out when ROI sizes differ. To be tested.\nNote to revert to the previous functionality generating individual images simply enable the disabled cases of the 3 yellow structures."
                            n35 = To Unsigned Long Integer(number=w163) -> (unsigned 32bit integer=w171:u32[][])
                            n36 = call "IMAQ ArrayToColorImage"("Image Pixels (U32)"=w171, "Image"=w168, "error in (no error)"=w167) -> ("Image Out"=w172:T26, "error out"=w170:errorcluster)  [unwired: 1 in, 1 out]
                            n37 = call "IMAQ AVI2 Write Frame"("error in (no error)"=w170, "Image"=w172, "AVI Refnum"=w169) -> ("error out"=w166:errorcluster, "Image Out (duplicate)"=w164:T26, "AVI Refnum (duplicate)"=w165:T27)  [unwired: 6 in]
                          }
                        }
                      }
                    }
                    n38 = disable-structure "Diagram Disable Structure" shown="Enabled" {
                      disable-tunnel: w78 -> [w92 _]
                      disable-tunnel: w81 -> [w91 _]
                      disable-tunnel: w79 -> [w90 _]
                      frame Enabled {
                        n39 = call "IMAQ AVI2 Close"("error in (no error)"=w91, "AVI Refnum"=w92) -> ()  [unwired: 9 in, 1 out]
                        n40 = call "IMAQ Dispose"("Image"=w90) -> ()  [unwired: 5 in, 1 out]
                      }
                      frame Disabled {
                      }
                    }
                    n41 = call "IMAQ Dispose"("Image"=w80, "error in (no error)"=w81) -> ("error out"=w69:errorcluster)  [unwired: 4 in]
                    n42 = flat-sequence {
                      tunnel: w69 -> [w83]
                      tunnel: [w83] -> w68
                      frame #0 {
                        n43 = Request Deallocation(TRUE ("flag")) -> ()
                      }
                    }
                  }
                  frame Error {
                  }
                }
              }
              frame Enabled {
                # "The execution speed of this code is not too important as it is run after data acquisition to post-process the TDMS data and pack it into AVI video files which are easier to handle than thousands of individual image files (previously)."
                n44 = case shown="No Error" w182 {
                  selector: w182 -> [_ w399]
                  tunnel: [w202 w399] -> w186
                  tunnel: w180 -> [w210 _]
                  tunnel: w183 -> [_ _]
                  tunnel: w178 -> [w199 _]
                  tunnel: w185 -> [w203 _]
                  tunnel: w184 -> [w190 _]
                  tunnel: w179 -> [w201 _]
                  tunnel: w181 -> [w200 _]
                  tunnel: w177 -> [w198 _]
                  tunnel: w175 -> [w196 _]
                  tunnel: w176 -> [w195 _]
                  tunnel: w174 -> [w188 _]
                  frame No Error {
                    # "Index of start cycle"
                    n45 = Decrement(x=w196) -> (x-1=w194:i32)
                    n46 = case shown="\"One multi-page TIFF file for each rectangle\"" w188 {
                      tunnel: w190 -> [w212 w215]
                      tunnel: [w211 w214] -> w189
                      frame "One multi-page TIFF file for each rectangle" {
                        w213 = T25 7 items=["Grayscale (U8)", "Grayscale (I16)", "Grayscale (SGL)", "Complex (CSG)", "RGB (U32)", "HSL (U32)", "RGB (U64)", "Grayscale (U16)"] ("Image Type")
                        n47 = call "IMAQ Create"("Image Name"=w212, "Image Type"=w213) -> ("New Image"=w211:T26)  [unwired: 3 in, 1 out]
                      }
                      frame "Individual TIFF files" {
                        w216 = T25 1 items=["Grayscale (U8)", "Grayscale (I16)", "Grayscale (SGL)", "Complex (CSG)", "RGB (U32)", "HSL (U32)", "RGB (U64)", "Grayscale (U16)"] ("Image Type")
                        n48 = call "IMAQ Create"("Image Name"=w215, "Image Type"=w216) -> ("New Image"=w214:T26)  [unwired: 3 in, 1 out]
                      }
                    }
                    n49 = Unbundle By Name(w199) -> ("Number of cycles"=w191:i32)
                    n50 = Unbundle By Name(w199) -> ("number of planes"=w204:i32)
                    n51 = disable-structure shown="Disabled" {
                      disable-tunnel: [w221 _] -> w207
                      disable-tunnel: [w220 _] -> w206
                      disable-tunnel: [w219 _] -> w205
                      disable-tunnel: w203 -> [w218 _]
                      disable-tunnel: w200 -> [w217 _]
                      frame Disabled {
                        n52 = call "Volume acq videos-Initialise.vi"("Channel"=w217, "created path"=w218) -> ("error out"=w219:errorcluster, "Temp Image"=w220:T26, "Refnum out"=w221:T27)  [unwired: 7 in]
                      }
                      frame Enabled {
                      }
                    }
                    n53 = Multiply(x=w191, y=w194) -> (x*y=w197:i32)
                    n54 = for {
                      N: w191 -> [_]
                      tunnel: w189 -> [w254]
                      tunnel: w203 -> [w253]
                      tunnel: w204 -> [w252]
                      tunnel: w206 -> [w251]
                      tunnel: w207 -> [w250]
                      tunnel: w205 -> [w249]
                      tunnel: [w233] -> w193
                      tunnel: [w248] -> w208
                      tunnel: [w247] -> w209
                      tunnel: w210 -> [w246]
                      tunnel: w190 -> [w245]
                      tunnel: w201 -> [w244]
                      tunnel: w199 -> [w242]
                      tunnel: w198 -> [w241]
                      tunnel: w197 -> [w238]
                      tunnel: w195 -> [w237]
                      tunnel: w188 -> [w234]
                      shift-right: [FALSE] -> _
                      shift-left: TRUE -> [w232]
                      i -> [w239]
                      stop <- w236 stop-if-true
                      # "FOR each functional acquisition cycle"
                      n55 = Add(x=w239, y=w238) -> (x+y=w240:i32)
                      n56 = call "Index volume data.vi"("Cycle index"=w239, "Single trial data (single channel)"=w241, "Parameters Cluster"=w242) -> ("3D"=w243:u16[][][])  [unwired: 5 in, 3 out]
                      n57 = for {
                        tunnel: w243 -> [w256] mode=indexing
                        tunnel: w254 -> [w276]
                        tunnel: w253 -> [w275]
                        tunnel: w252 -> [w261]
                        tunnel: w251 -> [w273]
                        tunnel: w250 -> [w274]
                        tunnel: w249 -> [w272]
                        tunnel: [w271] -> w233
                        tunnel: [w270] -> w248
                        tunnel: [w269] -> w247
                        tunnel: w246 -> [w265]
                        tunnel: w245 -> [w267]
                        tunnel: w244 -> [w266]
                        tunnel: w240 -> [w263]
                        tunnel: w237 -> [w259]
                        tunnel: w234 -> [w258]
                        tunnel: w232 -> [w255]
                        i -> [w262]
                        stop <- w260 stop-if-true
                        # "For each image/plane in a volume (or in a series of volumes) or for each rectangle when patches used. It adds a TIFF page to the multi-page TIFF file."
                        n58 = call <userlib>:"Calculate loop time.vi"() -> ("Loop time (ms)"=→"Loop time (ms)":u32)  [unwired: 11 in]
                        n59 = Index Array(array=w265, index=w262) -> (element=w264:dbl)
                        n60 = Equal To 0?(x=w264) -> (x = 0?=w268:bool)
                        n61 = case shown="\"One multi-page TIFF file for each rectangle\"" w258 {
                          tunnel: w276 -> [w293 w332]
                          tunnel: w275 -> [w292 _]
                          tunnel: w274 -> [w291 _]
                          tunnel: w273 -> [w290 _]
                          tunnel: w272 -> [w289 w333]
                          tunnel: [w288 w328] -> w271
                          tunnel: [w287 _] -> w270
                          tunnel: [w286 w332] -> w269
                          tunnel: w268 -> [w285 w329]
                          tunnel: w267 -> [w284 w331]
                          tunnel: w266 -> [w283 w327]
                          tunnel: w256 -> [w282 w334]
                          tunnel: w263 -> [w281 w335]
                          tunnel: w262 -> [w280 w330]
                          tunnel: w261 -> [w279 _]
                          tunnel: [w278 w337] -> w260
                          tunnel: w259 -> [w277 w336]
                          tunnel: w255 -> [_ w326]
                          frame "Individual TIFF files", Default {
                            n62 = disable-structure shown="Enabled" {
                              disable-tunnel: w293 -> [w294 _]
                              disable-tunnel: w292 -> [w307 _]
                              disable-tunnel: w279 -> [w312 _]
                              disable-tunnel: w280 -> [w311 _]
                              disable-tunnel: w291 -> [_ w322]
                              disable-tunnel: w290 -> [_ w321]
                              disable-tunnel: w289 -> [w297 w320]
                              disable-tunnel: [w303 w319] -> w288
                              disable-tunnel: [_ w318] -> w287
                              disable-tunnel: [w294 w317] -> w286
                              disable-tunnel: w285 -> [w296 _]
                              disable-tunnel: w282 -> [w295 w316]
                              disable-tunnel: w284 -> [w310 _]
                              disable-tunnel: w283 -> [w309 _]
                              disable-tunnel: w280 -> [w302 _]
                              disable-tunnel: w281 -> [w306 _]
                              disable-tunnel: [w304 _] -> w278
                              disable-tunnel: w277 -> [_ _]
                              frame Enabled {
                                n63 = Index Array(array=w307, index=w302) -> (element=w308:path)
                                n64 = disable-structure shown="Enabled" {
                                disable-tunnel: w295 -> [w315 _]
                                frame Disabled {
                                n65 = call "AVI Video Save.vi"("Image Pixels"=w315) -> ()  [unwired: 9 in, 2 out]
                                }
                                frame Enabled {
                                }
                                }
                                n66 = call "Funct TIFF export-Generate image from data.vi"("Horisontal (T)"=w296, "3D"=w295, "error in (no error)"=w297, "Rectangle index"=w311, "Image Name"=w310, "Refnum in"=w294) -> ("error out"=w313:errorcluster, "Refnum out"=w314:T26)  [unwired: 4 in]
                                n67 = call "Generate volume image path.vi"("Channel to process"=w309, "Volume index"=0, "Number of planes"=w312, "Plane index (within its volume)"=w306, "Folder path"=w308) -> ("File path"=w299:path)  [unwired: 5 in, 1 out]
                                n68 = global read "gl_funct TIFF export globals.vi" "Stop TIFF export"() -> (w305:bool)
                                n69 = call-poly "IMAQ Write File 2"("error in (no error)"=w313, "File Path"=w299, "Image"=w314) -> ("error out"=w301:errorcluster, "Image Out (duplicate)"=w300:T26)  [unwired: 7 in]
                                n70 = call "IMAQ Dispose"("Image"=w300, "error in (no error)"=w301) -> ("error out"=w303:errorcluster)  [unwired: 4 in]
                                n71 = Compound Arithmetic op=OR(w303, w305) -> (w304:bool)
                              }
                              frame Disabled {
                                # "WARNING!\nPotential issues with this basic implementation can be as follows:\n\n1. It uses the AVI2 implementation which doesn't support generating videos >2GB. \nThe logic would need to be upgraded similarly to the timelapse imaging code to split the recording into multiple AVI files of <2GB and named suitable.\n\n2. It will place all recorded images in the same AVI file even when they belong to different ROIs like different volumes or different squares.\n\n3. It may error out when ROI sizes differ. To be tested.\nNote to revert to the previous functionality generating individual images simply enable the disabled cases of the 3 yellow structures."
                                n72 = To Unsigned Long Integer(number=w316) -> (unsigned 32bit integer=w324:u32[][])
                                n73 = call "IMAQ ArrayToColorImage"("Image Pixels (U32)"=w324, "Image"=w321, "error in (no error)"=w320) -> ("Image Out"=w325:T26, "error out"=w323:errorcluster)  [unwired: 1 in, 1 out]
                                n74 = call "IMAQ AVI2 Write Frame"("error in (no error)"=w323, "Image"=w325, "AVI Refnum"=w322) -> ("error out"=w319:errorcluster, "Image Out (duplicate)"=w317:T26, "AVI Refnum (duplicate)"=w318:T27)  [unwired: 6 in]
                              }
                            }
                          }
                          frame "One multi-page TIFF file for each rectangle" {
                            n75 = disable-structure shown="TARGET_BITNESS==32, Default" {
                              disable-tunnel: [w358 _] -> w337
                              disable-tunnel: w336 -> [w357 _]
                              disable-tunnel: w335 -> [w351 _]
                              disable-tunnel: w334 -> [w350 _]
                              disable-tunnel: w333 -> [w345 _]
                              disable-tunnel: w332 -> [w344 _]
                              disable-tunnel: w331 -> [w343 _]
                              disable-tunnel: w330 -> [w342 _]
                              disable-tunnel: w329 -> [w341 _]
                              disable-tunnel: [w340 _] -> w328
                              disable-tunnel: w327 -> [w339 _]
                              disable-tunnel: w326 -> [w338 _]
                              frame condition #0 {
                                n76 = case shown="False" w341 {
                                tunnel: w350 -> [w397 w398]
                                tunnel: [w396 w398] -> w356
                                frame False {
                                # "Vertical"
                                n77 = Transpose 2D Array(2D array=w397) -> (transposed array=w396:u16[][])
                                }
                                frame True {
                                # "Horisontal"
                                }
                                }
                                n78 = Increment(x=w351) -> (x+1=w348:i32)
                                n79 = disable-structure shown="Enabled" {
                                disable-tunnel: [w394 "" ("ImageDescription")] -> w352
                                frame Disabled {
                                w394 = "OME.xml.string"  # ImageDescription
                                }
                                frame Enabled {
                                }
                                }
                                n80 = Array Size(array=w356) -> (size(s)=w355:i32[])
                                n81 = Index Array(array=w357, index=w342) -> (element=w349:i32)
                                n82 = To Unsigned Long Integer(number=w348) -> (unsigned 32bit integer=w347:u32)
                                n83 = Index Array(array=w355) -> (element #1=w354:i32, element #2=w353:i32)  [unwired: 2 in]
                                n84 = disable-structure shown="Enabled" {
                                disable-tunnel: [w369 w371 w382 w390] -> w340
                                disable-tunnel: w356 -> [w368 w372 w385 w389]
                                disable-tunnel: w354 -> [w367 _ _ _]
                                disable-tunnel: w353 -> [w366 _ _ _]
                                disable-tunnel: w352 -> [w365 _ _ _]
                                disable-tunnel: w349 -> [w364 w377 w383 w392]
                                disable-tunnel: w348 -> [w363 w378 w384 w393]
                                disable-tunnel: w347 -> [w362 w376 w379 w391]
                                disable-tunnel: w345 -> [w361 w373 w386 w388]
                                disable-tunnel: w344 -> [_ w375 w387 _]
                                disable-tunnel: w343 -> [_ _ _ _]
                                disable-tunnel: w342 -> [_ _ _ _]
                                disable-tunnel: w339 -> [w360 _ _ _]
                                disable-tunnel: w338 -> [w359 _ _ _]
                                frame Enabled {
                                # "Trial 1 = 20 sec\nTrial 2 = 40 sec\nTrial 3 = 65 sec\nTrial 4 = 90 sec\nTrial 5 = 130 sec\nTrial 6 = 155 sec"
                                # "Fastest"
                                # "Generated 1.75MB per trial"
                                # "Write line by line"
                                n85 = call "libtiff3_write_tiff page 16bit.vi"("Handle"=w364, "Image Pixels (U16)"=w368, "Reset"=w359, "Channel to process"=w360, "ImageDescription"=w365, "error in (no error)"=w361, "page"=w362, "x.pixels"=w366, "totalpages"=w363, "y.pixels"=w367) -> ("error out"=w369:errorcluster)  [unwired: 8 in, 1 out]
                                }
                                frame Disabled {
                                # "Trial 1 = 35 sec\nTrial 2 = 60 sec\nTrial 3 = 85 sec"
                                # "Slow"
                                # "Generated 16.69MB per trial"
                                # "Write strips"
                                n86 = call "IMAQ ArrayToImage"("Image Pixels (U16)"=w372, "error in (no error)"=w373, "Image"=w375) -> ("error out"=w374:errorcluster, "Image Out"=w370:T26)  [unwired: 7 in]
                                n87 = call "libtiff3 write StripedPage raw U16-mod.vi"("totalpages"=w378, "error in (no error)"=w374, "page"=w376, "Image"=w370, "Handle"=w377) -> ("error out"=w371:errorcluster)  [unwired: 5 in, 1 out]
                                }
                                frame Disabled {
                                # "Slow"
                                # "Trial 1 = 22 sec\nTrial 2 = 45 sec\nTrial 3 = 80 sec"
                                # "Generated 16.69MB per trial"
                                # "Write raw strips"
                                n88 = call "IMAQ ArrayToImage"("Image Pixels (U16)"=w385, "error in (no error)"=w386, "Image"=w387) -> ("error out"=w381:errorcluster, "Image Out"=w380:T26)  [unwired: 7 in]
                                n89 = call "libtiff3 write StripedPage raw U16-mod.vi"("totalpages"=w384, "error in (no error)"=w381, "page"=w379, "Image"=w380, "Handle"=w383) -> ("error out"=w382:errorcluster)  [unwired: 5 in, 1 out]
                                }
                                frame Disabled {
                                # "My stripped down\ncustom VI."
                                # "Trial 1 = 15 sec\nTrial 2 = 40 sec\nTrial 3 = 66 sec\nTrial 4 = 91 sec"
                                # "Generated 16.69MB per trial"
                                # "Writes raw strips"
                                n90 = call "Funct TIFF export-Custom Write multi-page TIFF.vi"("Image Pixels (U16)"=w389, "totalpages"=w393, "error in (no error)"=w388, "page"=w391, "Handle"=w392) -> ("error out"=w390:errorcluster)  [unwired: 5 in, 1 out]
                                }
                                }
                                n91 = global read "gl_funct TIFF export globals.vi" "Stop TIFF export"() -> (w346:bool)
                                n92 = Compound Arithmetic op=OR(w340, w346) -> (w358:bool)
                              }
                              frame condition #1 (active) {
                              }
                            }
                          }
                        }
                      }
                      n93 = global read "gl_funct TIFF export globals.vi" "Stop TIFF export"() -> (w235:bool)
                      n94 = Compound Arithmetic op=OR(w233, w235) -> (w236:bool)
                    }
                    n95 = disable-structure "Diagram Disable Structure" shown="Enabled" {
                      disable-tunnel: w208 -> [w227 _]
                      disable-tunnel: w193 -> [w224 w229]
                      disable-tunnel: w209 -> [w226 w230]
                      disable-tunnel: [w225 w228] -> w192
                      frame Disabled {
                        n96 = call "IMAQ AVI2 Close"("error in (no error)"=w224, "AVI Refnum"=w227) -> ()  [unwired: 9 in, 1 out]
                        n97 = call "IMAQ Dispose"("Image"=w226, "error in (no error)"=w224) -> ("error out"=w225:errorcluster)  [unwired: 4 in]
                      }
                      frame Enabled {
                        n98 = call "IMAQ Dispose"("Image"=w230, "error in (no error)"=w229) -> ("error out"=w228:errorcluster)  [unwired: 4 in]
                      }
                    }
                    n99 = flat-sequence {
                      tunnel: w192 -> [w222]
                      tunnel: [w222] -> w202
                      frame #0 {
                        n100 = Request Deallocation(TRUE ("flag")) -> ()
                      }
                    }
                  }
                  frame Error {
                  }
                }
              }
            }
          }
        }
        frame Disabled {
          # "The While Loop causes all instances of this VI to execute in parallel. (While loop is REDUNDANT)"
          n101 = while {
            tunnel: [w425] -> w411
            tunnel: w410 -> [w424]
            tunnel: w407 -> [w414]
            tunnel: w409 -> [w421]
            tunnel: w405 -> [w418]
            tunnel: w408 -> [w415]
            tunnel: w406 -> [w413]
            tunnel: [w412] -> w404
            stop <- TRUE stop-if-true
            # "The execution speed of this code is not too important as it is run after data acquisition to post-process the TDMS data and pack it into AVI video files which are easier to handle than thousands of individual image files (previously)."
            n102 = call "Reshape volume imaging data.vi"("tdms file ref"=w413, "TDMS file path & name"=w414, "All header parameters"=w418, "error in (no error)"=w421, "Channel to process"=w415) -> ("tdms file out"=w412:refnum<k34>, "Volumetric parameters"=w416:T24, "Angles (deg)"=w417:dbl[], "error out"=w422:errorcluster)  [unwired: 5 in, 2 out]
            n103 = case shown="\"Green\"" w415 {
              tunnel: ["Red" ("Image Name") "Green" ("Image Name")] -> w423
              tunnel: [Channel_Selector."Red Channel" ("Channel") Channel_Selector."Green Channel" ("Channel")] -> w420
              frame "Red", Default {
                # "Red"
              }
              frame "Green" {
                # "Green"
              }
            }
            n104 = case shown="No Error" w422 {
              selector: w422 -> [_ w538]
              tunnel: [w432 w538] -> w425
              tunnel: w417 -> [w447 _]
              tunnel: w412 -> [w439 _]
              tunnel: w416 -> [w436 _]
              tunnel: w424 -> [w435 _]
              tunnel: w423 -> [w434 _]
              tunnel: w415 -> [w431 _]
              tunnel: w420 -> [w430 _]
              frame No Error {
                w438 = T25 1 items=["Grayscale (U8)", "Grayscale (I16)", "Grayscale (SGL)", "Complex (CSG)", "RGB (U32)", "HSL (U32)", "RGB (U64)", "Grayscale (U16)"] ("Image Type")
                n105 = disable-structure "Diagram Disable Structure" shown="Enabled" {
                  disable-tunnel: [w454 _] -> w440
                  disable-tunnel: [w453 _] -> w441
                  disable-tunnel: [w452 _] -> w442
                  disable-tunnel: w435 -> [w451 _]
                  disable-tunnel: w430 -> [w450 _]
                  frame Enabled {
                    n106 = call "Volume acq videos-Initialise.vi"("Channel"=w450, "created path"=w451) -> ("error out"=w454:errorcluster, "Temp Image"=w453:T26, "Refnum out"=w452:T27)  [unwired: 7 in]
                  }
                  frame Disabled {
                  }
                }
                n107 = Unbundle By Name(w436) -> ("number of planes"=w437:i32)
                n108 = call "IMAQ Create"("Image Name"=w434, "Image Type"=w438) -> ("New Image"=w445:T26)  [unwired: 3 in, 1 out]
                n109 = for {
                  tunnel: w439 -> [w471]
                  tunnel: w445 -> [w470]
                  tunnel: w435 -> [w469] mode=indexing
                  tunnel: w437 -> [w467]
                  tunnel: w441 -> [w466]
                  tunnel: w442 -> [w465]
                  tunnel: w440 -> [w464]
                  tunnel: [w463] -> w446
                  tunnel: [w462] -> w443
                  tunnel: [w461] -> w444
                  tunnel: w447 -> [w460]
                  tunnel: w434 -> [w459]
                  tunnel: w431 -> [w458]
                  i -> [w468]
                  # "For each volume in the sequence / Or for each cycle during funct ack."
                  n110 = for {
                    tunnel: w471 -> [w475]
                    tunnel: w470 -> [w488]
                    tunnel: w469 -> [w487]
                    tunnel: w468 -> [w486]
                    tunnel: w467 -> [w485]
                    tunnel: w466 -> [w483]
                    tunnel: w465 -> [w484]
                    tunnel: w464 -> [w482]
                    tunnel: [w481] -> w463
                    tunnel: [w480] -> w462
                    tunnel: [w479] -> w461
                    tunnel: w460 -> [w474]
                    tunnel: w459 -> [w477]
                    tunnel: w458 -> [w476]
                    i -> [w473]
                    # "For each image/plane in a volume or each rectangle if funct ack."
                    n111 = Index Array(array=w474, index=w473) -> (element=w472:dbl)
                    n112 = Equal To 0?(x=w472) -> (x = 0?=w478:bool)
                    n113 = disable-structure shown="Disabled" {
                      disable-tunnel: w488 -> [w505 _]
                      disable-tunnel: w487 -> [w500 _]
                      disable-tunnel: w486 -> [w498 _]
                      disable-tunnel: w485 -> [w497 _]
                      disable-tunnel: w473 -> [w496 _]
                      disable-tunnel: w484 -> [_ w534]
                      disable-tunnel: w483 -> [_ w533]
                      disable-tunnel: w482 -> [_ w532]
                      disable-tunnel: [_ w531] -> w481
                      disable-tunnel: [_ w530] -> w480
                      disable-tunnel: [_ w529] -> w479
                      disable-tunnel: w478 -> [w495 _]
                      disable-tunnel: w475 -> [w490 w528]
                      disable-tunnel: w477 -> [w493 _]
                      disable-tunnel: w476 -> [w489 _]
                      frame Disabled {
                        # "WARNING!\nUpgrade this code to generate AVI video files instead of individual images.\nUse the code in the \"AVI U16 write-read multi frame.vi\" in C:\\UCL\\RIG 3\\Source Code\\Prototyping\\AVI saves prototyping."
                        n114 = case shown="True" w495 {
                          tunnel: w490 -> [w507 w508]
                          tunnel: [w506 w508] -> w494
                          frame False {
                            # "Vertical"
                            n115 = Transpose 2D Array(2D array=w507) -> (transposed array=w506:refnum<k34>[][])
                          }
                          frame True {
                            # "Horisontal"
                          }
                        }
                        n116 = call "AVI Video Save.vi"("Image Pixels"=w490) -> ()  [unwired: 9 in, 2 out]
                        n117 = call "IMAQ ArrayToImage"("Image Pixels (I16)"=w494, "Image"=w505) -> ("error out"=w501:errorcluster, "Image Out"=w504:T26)  [unwired: 8 in]
                        n118 = Concatenate Strings(w493, "1" ("string")) -> (w491:string)
                        n119 = call "Generate volume image path.vi"("Channel to process"=w489, "Volume index"=w498, "Number of planes"=w497, "Plane index (within its volume)"=w496, "Folder path"=w500) -> ("File path"=w499:path)  [unwired: 5 in, 1 out]
                        n120 = disable-structure shown="Enabled" {
                          disable-tunnel: w496 -> [w519 _]
                          disable-tunnel: w504 -> [w518 w527]
                          disable-tunnel: [w517 w527] -> w503
                          disable-tunnel: [w515 w526] -> w502
                          disable-tunnel: w501 -> [w516 w526]
                          disable-tunnel: w491 -> [w514 _]
                          frame Enabled {
                            w521 = T25 1 items=["Grayscale (U8)", "Grayscale (I16)", "Grayscale (SGL)", "Complex (CSG)", "RGB (U32)", "HSL (U32)", "RGB (U64)"] ("Image Type")
                            # "Warning!\n-32767 or -32768??"
                            n121 = Number To Decimal String(number=w519) -> (decimal integer string=w522:string)  [unwired: 1 in]
                            n122 = Concatenate Strings(w514, w522) -> (w523:string)
                            n123 = call "IMAQ Create"("Image Name"=w523, "Image Type"=w521, "error in (no error)"=w516) -> ("New Image"=w524:T26, "error out"=w525:errorcluster)  [unwired: 2 in]
                            n124 = call "IMAQ Add"("Image Src A"=w518, "Constant"=i16 -32768, "Image Dst"=w524, "error in (no error)"=w525) -> ("Image Dst Out"=w517:T26, "error out"=w515:errorcluster)  [unwired: 3 in]
                          }
                          frame Disabled {
                          }
                        }
                        n125 = disable-structure shown="Enabled" {
                          disable-tunnel: w503 -> [w511 _]
                          disable-tunnel: w502 -> [w510 _]
                          disable-tunnel: w499 -> [w509 _]
                          frame Enabled {
                            n126 = call-poly "IMAQ Write File 2"("error in (no error)"=w510, "File Path"=w509, "Image"=w511) -> ("error out"=w513:errorcluster, "Image Out (duplicate)"=w512:T26)  [unwired: 7 in]
                            n127 = call "IMAQ Dispose"("Image"=w512, "error in (no error)"=w513) -> ()  [unwired: 4 in, 1 out]
                          }
                          frame Disabled {
                          }
                        }
                      }
                      frame Enabled {
                        # "WARNING!\nPotential issues with this basic implementation can be as follows:\n\n1. It uses the AVI2 implementation which doesn't support generating videos >2GB. \nThe logic would need to be upgraded similarly to the timelapse imaging code to split the recording into multiple AVI files of <2GB and named suitable.\n\n2. It will place all recorded images in the same AVI file even when they belong to different ROIs like different volumes or different squares.\n\n3. It may error out when ROI sizes differ. To be tested.\nNote to revert to the previous functionality generating individual images simply enable the disabled cases of the 3 yellow structures."
                        n128 = To Unsigned Long Integer(number=w528) -> (unsigned 32bit integer=w536:u32)
                        n129 = call "IMAQ ArrayToColorImage"("Image Pixels (U32)"=w536, "Image"=w533, "error in (no error)"=w532) -> ("Image Out"=w537:T26, "error out"=w535:errorcluster)  [unwired: 1 in, 1 out]
                        n130 = call "IMAQ AVI2 Write Frame"("error in (no error)"=w535, "Image"=w537, "AVI Refnum"=w534) -> ("error out"=w531:errorcluster, "Image Out (duplicate)"=w529:T26, "AVI Refnum (duplicate)"=w530:T27)  [unwired: 6 in]
                      }
                    }
                  }
                }
                n131 = disable-structure "Diagram Disable Structure" shown="Enabled" {
                  disable-tunnel: w443 -> [w457 _]
                  disable-tunnel: w446 -> [w456 _]
                  disable-tunnel: w444 -> [w455 _]
                  frame Enabled {
                    n132 = call "IMAQ AVI2 Close"("error in (no error)"=w456, "AVI Refnum"=w457) -> ()  [unwired: 9 in, 1 out]
                    n133 = call "IMAQ Dispose"("Image"=w455) -> ()  [unwired: 5 in, 1 out]
                  }
                  frame Disabled {
                  }
                }
                n134 = call "IMAQ Dispose"("Image"=w445, "error in (no error)"=w446) -> ("error out"=w433:errorcluster)  [unwired: 4 in]
                n135 = flat-sequence {
                  tunnel: w433 -> [w448]
                  tunnel: [w448] -> w432
                  frame #0 {
                    n136 = Request Deallocation(TRUE ("flag")) -> ()
                  }
                }
              }
              frame Error {
              }
            }
          }
        }
      }
    }
    frame True {
    }
  }
  "error out" <- w14
  "tdms file out" <- w1
